vi "Transfer Function (DBL Array).vi"(2 "initialize":bool, 3 "dt":dbl=1e-09 min=1e-09 format="%.6f", 4 "Transfer functions":T1(array[cluster])=[{"numerator"=[], "denominator"=[]}] {"denominator" format="%.2f"; "numerator" format="%.2f"}, 5 "input points":dbl[](array[numeric]) format="%.2f") -> (1 "output points":dbl[](array[numeric]) format="%.2f")   [LabVIEW 2017, in "NI_AdvCtrl_continuous linear.lvlib"]
doc: "LabVIEW no longer supports this VI. You can obtain similar functionality by installing the LabVIEW Simulation Module.\n\nCalculates the new output, where the transfer function and the input are given. The transfer function is described by two polynomials, numerator(s) and denominator(s)."
uses:
  <vilib>/addons/control/advanced/NI_AdvCtrl_continuous linear.lvlib
panel:
  # "t"
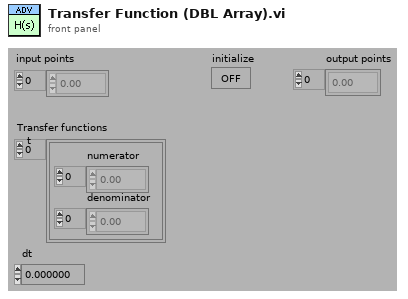
[diagram p1: front panel]
types:
  T1 = cluster{"numerator":dbl[], "denominator":dbl[]}[]
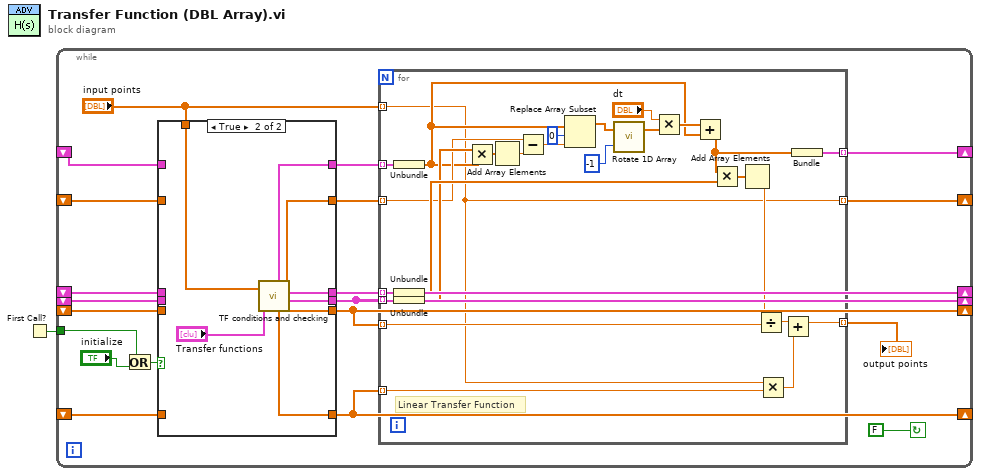
[diagram p0: block diagram]
diagram:
  n1 = First Call?() -> (First Call?: T/F=w1:bool)
  n2 = while {
    shift-left: _ -> [w7]
    shift-right: [w8] -> _
    shift-left: _ -> [w13]
    shift-right: [w10] -> _
    tunnel: w1 -> [w14]
    shift-left: _ -> [w18]
    shift-right: [w2] -> _
    shift-left: _ -> [w19]
    shift-right: [w17] -> _
    shift-left: _ -> [w20]
    shift-right: [w11] -> _
    shift-left: _ -> [w21]
    shift-right: [w4] -> _
    stop <- FALSE continue-if-true
    n3 = Or(x=w14, y="initialize") -> (x .or. y?=w3:bool)
    n4 = case shown="True" w3 {
      tunnel: [w50 w54] -> w2
      tunnel: [w51 w61] -> w17
      tunnel: [w53 w60] -> w4
      tunnel: [w52 w59] -> w11
      tunnel: w21 -> [w53 _]
      tunnel: w20 -> [w52 _]
      tunnel: w19 -> [w51 _]
      tunnel: w18 -> [w50 _]
      tunnel: [w49 w57] -> w12
      tunnel: w13 -> [w49 _]
      tunnel: w7 -> [w48 _]
      tunnel: [w48 w55] -> w6
      tunnel: "input points" -> [_ w56]
      frame False {
      }
      frame True {
        n5 = call <vilib>:"TF conditions and checking.vi"("Input Points"=w56, "Transfer Functions"="Transfer functions") -> ("internal states"=w57:cluster{dbl[]}[], "additive constants"=w54:dbl[], "previous samples"=w55:dbl[], "numerators"=w60:cluster{"Numerator new":dbl[]}[], "denominators"=w59:cluster{dbl[]}[], "gains"=w61:dbl[])
      }
    }
    n6 = for {
      tunnel: w2 -> [w27] mode=indexing
      tunnel: w17 -> [w47] mode=indexing
      tunnel: w12 -> [w41] mode=indexing
      tunnel: w11 -> [w40] mode=indexing
      tunnel: [w36] -> w10 mode=indexing
      tunnel: w4 -> [w37] mode=indexing
      tunnel: "input points" -> [w26] mode=indexing
      tunnel: [w29] -> w9 mode=indexing
      tunnel: [w26] -> w8 mode=indexing
      tunnel: w6 -> [w33] mode=indexing
      # "Linear Transfer Function"
      n7 = Unbundle(w41) -> (w31:dbl[])
      n8 = Unbundle(w37) -> ("Numerator new"=w35:dbl[])
      n9 = Unbundle(w40) -> (w34:dbl[])
      n10 = Multiply(x=w34, y=w31) -> (x*y=w44:dbl[])
      n11 = Add Array Elements(numeric array=w44) -> (sum=w43:dbl)
      n12 = Subtract(x=w33, y=w43) -> (x-y=w46:dbl)
      n13 = Replace Array Subset(array=w31, new element=w46, index=0 ("Index")) -> (w25:dbl[])
      n14 = call <vilib>:"Rotate 1D Array.vi"("n"=-1, "array"=w25) -> ("array (last n elements first)"=w24:dbl[])  [unwired: 1 out]
      n15 = Multiply(x="dt", y=w24) -> (x*y=w42:dbl[])
      n16 = Add(x=w42, y=w31) -> (x+y=w38:dbl[])
      n17 = Multiply(x=w38, y=w35) -> (x*y=w39:dbl[])
      n18 = Add Array Elements(numeric array=w39) -> (sum=w32:dbl)
      n19 = Divide(x=w32, y=w47) -> (x/y=w30:dbl)
      n20 = Multiply(x=w26, y=w27) -> (x*y=w28:dbl)
      n21 = Add(x=w30, y=w28) -> (x+y=w29:dbl)
      n22 = Bundle(w38) -> (w36:cluster{dbl[]})  [unwired: 1 in]
    }
    "output points" <- w9
  }
